vi "edittest parse POST step config.vi"(8 "error in (no error)":errorcluster, 9 "POST (empty)":T2, 10 "sxSequenceId (\"\")":string, 11 "Connection Refnum":T1) -> (0 "error out":errorcluster, 2 "Step Record":T3, 3 "dup Connection Refnum":T1)   [LabVIEW 2011]
uses:
  server/database/Steps/Step Record.ctl
  ITK EXT/utils/keyedarr.llb/Keyed Array.ctl
  Summitek EXT/ODBC/SQL Controls/Connection Refnum.ctl
  ITK EXT/utils/strutil.llb/Case Matching.ctl
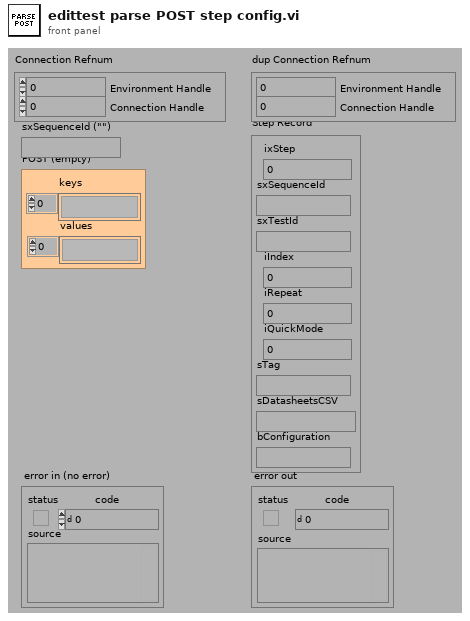
[diagram p1: front panel]
types:
  T1 = typedef "Connection Refnum.ctl" = cluster{"Environment Handle":i32, "Connection Handle":i32}
  T2 = typedef "Keyed Array.ctl" = cluster{"keys":string[], "values":string[]}
  T3 = typedef "Step Record.ctl" = cluster{"ixStep":i32, "sxSequenceId":string, "sxTestId":string, "iIndex":i32, "iRepeat":i32, "iQuickMode":i32, "sTag":string, "sDatasheetsCSV":string, "bConfiguration":string}
  T4 = typedef "Case Matching.ctl" = enum16{"a != A", "a == A", "system"}
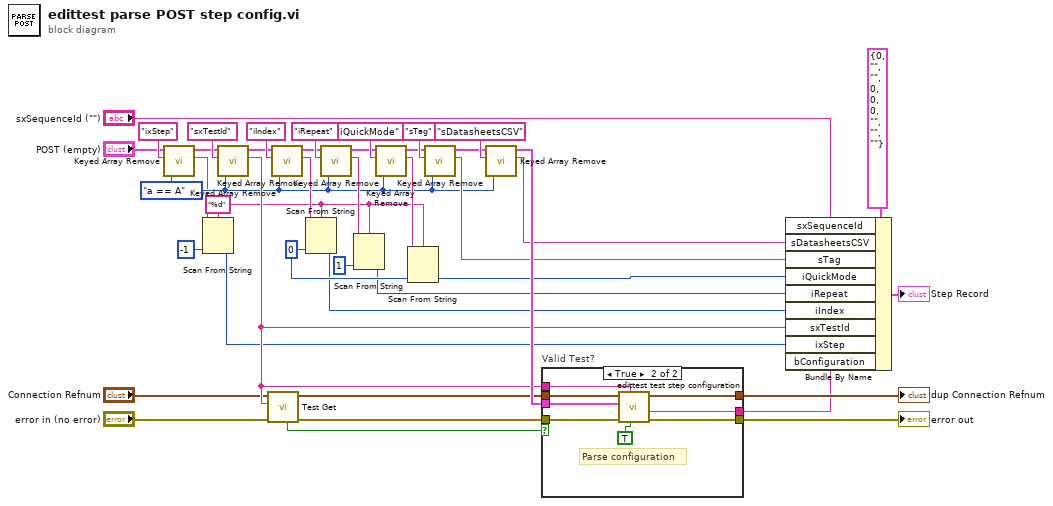
[diagram p0: block diagram]
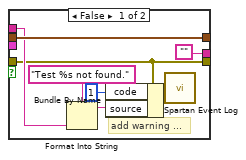
[diagram p2: hidden frame]
diagram:
  w3 = "%d" ("format string")
  w5 = Case_Matching."a == A" ("case matching (sensitive)")
  w17 = 0 ("default value 1")
  n1 = call "Keyed Array Remove.vi"("case matching (sensitive)"=w5, "key"="ixStep", "array in"="POST (empty)") -> ("value"=w2:string, "array out"=w6:T2)  [unwired: 3 out]
  n2 = Scan From String(format string=w3, input string=w2, default 1=-1 ("default value 1")) -> (output 1=w1:i32)  [unwired: 2 in, 3 out]
  n3 = call "Keyed Array Remove.vi"("case matching (sensitive)"=w5, "key"="sxTestId", "array in"=w6) -> ("value"=w11:string, "array out"=w23:T2)  [unwired: 3 out]
  n4 = call "Test Get.vi"("error in (no error)"="error in (no error)", "Test_ID"=w11, "Connection Refnum"="Connection Refnum") -> ("error out"=w31:errorcluster, "Connection Refnum"=w9:T1, "Data Present"=w24:bool)  [unwired: 6 out]
  n5 = call "Keyed Array Remove.vi"("case matching (sensitive)"=w5, "key"="iIndex", "array in"=w23) -> ("value"=w42:string, "array out"=w22:T2)  [unwired: 3 out]
  n6 = Scan From String(format string=w3, input string=w42, default 1=w17) -> (output 1=w12:i32)  [unwired: 2 in, 3 out]
  n7 = call "Keyed Array Remove.vi"("case matching (sensitive)"=w5, "key"="iRepeat", "array in"=w22) -> ("value"=w41:string, "array out"=w21:T2)  [unwired: 3 out]
  n8 = Scan From String(format string=w3, input string=w41, default 1=1 ("default value 1")) -> (output 1=w13:i32)  [unwired: 2 in, 3 out]
  n9 = call "Keyed Array Remove.vi"("case matching (sensitive)"=w5, "key"="iQuickMode", "array in"=w21) -> ("value"=w39:string, "array out"=w20:T2)  [unwired: 3 out]
  n10 = Scan From String(format string=w3, input string=w39, default 1=w17) -> (output 1=w14:i32)  [unwired: 2 in, 3 out]
  n11 = call "Keyed Array Remove.vi"("case matching (sensitive)"=w5, "key"="sTag", "array in"=w20) -> ("value"=w15:string, "array out"=w19:T2)  [unwired: 3 out]
  n12 = call "Keyed Array Remove.vi"("case matching (sensitive)"=w5, "key"="sDatasheetsCSV", "array in"=w19) -> ("value"=w16:string, "array out"=w18:T2)  [unwired: 2 in, 1 out]
  n13 = case "Valid Test?" shown="True" w24 {
    tunnel: w31 -> [w47 w58]
    tunnel: [w47 w57] -> w30
    tunnel: w9 -> [w50 w52]
    tunnel: [w50 w51] -> w28
    tunnel: w18 -> [_ w54]
    tunnel: ["" w55] -> w25
    tunnel: w11 -> [w48 w53]
    frame False {
      # "add warning ..."
      n14 = Format Into String(format string="Test %s not found.", w48) -> (resulting string=w45:string)  [unwired: 2 in, 1 out]
      n15 = Bundle By Name(cluster=w47, "code"=1, "source"=w45) -> (w46:errorcluster)
      n16 = call "Spartan Event Log.vi"("error in (no error)"=w46) -> ()  [unwired: 7 in, 1 out]
    }
    frame True {
      # "Parse configuration"
      n17 = call "edittest test step configuration.vi"("Write? (f)"=TRUE, "sxTestId (\"\")"=w53, "error in (no error)"=w58, "POSTed Step Config (to Write to bConfiguration)\nOR\nTemplate Keys (empty)"=w54, "Connection Refnum"=w52) -> ("error out"=w57:errorcluster, "bConfiguration"=w55:string, "Connection Refnum"=w51:T1)  [unwired: 2 in, 2 out]
    }
  }
  "error out" <- w30
  "dup Connection Refnum" <- w28
  n18 = Bundle By Name(cluster=T3 {"ixStep"=0, "sxSequenceId"="", "sxTestId"="", "iIndex"=0, "iRepeat"=0, "iQuickMode"=0, "sTag"="", "sDatasheetsCSV"="", "bConfiguration"=""} ("Step Record"), "sxSequenceId"="sxSequenceId (\"\")", "sDatasheetsCSV"=w16, "sTag"=w15, "iQuickMode"=w14, "iRepeat"=w13, "iIndex"=w12, "sxTestId"=w11, "ixStep"=w1, "bConfiguration"=w25) -> (→"Step Record":T3)
